vi "Action.vi"(8 "error in (no error)":errorcluster, 10 "OOQMH in":refnum<class "OOQMH.lvclass">, 11 "Set Polling Message in":refnum<class "Set Polling Message.lvclass">) -> (0 "error out":errorcluster, 2 "OOQMH out":refnum<class "OOQMH.lvclass">, 3 "Set Polling Message out":refnum<class "Set Polling Message.lvclass">)   [LabVIEW 2024, in "OOQMH.lvlib" / "Set Polling Message.lvclass"]
uses:
  Set Polling Message.lvclass
  OOQMH/OOQMH.lvclass
  Set Polling Message.lvclass/Set Polling Message.ctl
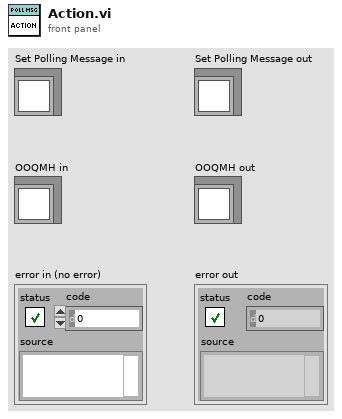
[diagram p1: front panel]
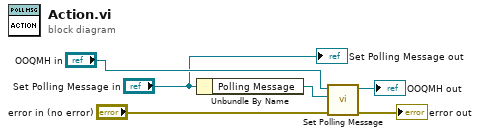
[diagram p0: block diagram]
diagram:
  n1 = Unbundle By Name("Set Polling Message in") -> ("Polling Message"=w1:refnum<class "Message.lvclass">)
  n2 = call-dynamic "Set Polling Message.vi"("error in (no error)"="error in (no error)", "Polling Message"=w1, "OOQMH in"="OOQMH in") -> ("error out"=→"error out":errorcluster, "OOQMH out"=→"OOQMH out":refnum<class "OOQMH.lvclass">)  [unwired: 7 in]
  "Set Polling Message out" <- "Set Polling Message in"
